vi "BeginTankDrive.vi"() -> (0 "error out":errorcluster)   [LabVIEW 2012]
uses:
  <vilib>/Rock Robotics/WPI/CAN/Jaguar/SubVIs/WPI_CANJaguar_SpeedReference.ctl
  <vilib>/Rock Robotics/WPI/CAN/Jaguar/SubVIs/WPI_CANJaguar_ControlMode.ctl
  <vilib>/Rock Robotics/WPI/MotorControl/WPI_MotorControlOpenCANJaguar.vi
  <vilib>/Rock Robotics/WPI/CAN/Jaguar/SubVIs/WPI_CANJaguar_BrakeCoastMode.ctl
panel:
  out "Succeeded?":bool
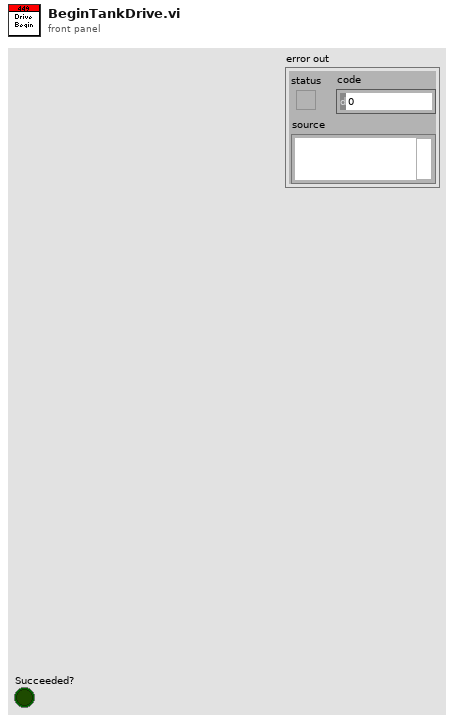
[diagram p1: front panel]
types:
  T1 = typedef "WPI_CANJaguar_ControlMode.ctl" = enum8{"Percent VBus", "Current", "Speed", "Position", "Voltage"}
  T2 = typedef "WPI_CANJaguar_SpeedReference.ctl" = u8
  T3 = typedef "WPI_MotorControlDeviceRef.ctl" = cluster{"DeviceStatus":errorcluster, "Type":enum16{"PWM", "CAN"}, "PWM":cluster{"Digital Module":T4, "PWM Channel":T5, "DeadBand":T6}, "CAN":cluster{"Device Number":u8, "Control Mode":T1, "Semaphore":T7, "Max Vout":dbl}, "Invert":bool, "TransformRef":T8, "InvTransformRef":T8}
  T4 = typedef "FPGA_TypedefDigitalModule.ctl" = enum16{"Digital Module 1", "Digital Module 2"}
  T5 = typedef "FPGA_DIOPWMChannel.ctl" = enum8{"PWM 1", "PWM 2", "PWM 3", "PWM 4", "PWM 5", "PWM 6", "PWM 7", "PWM 8", "PWM 9", "PWM 10", "Invalid"}
  T6 = typedef "WPI_PWMDeadband.ctl" = cluster{"Name":string, "maxPositivePwm":i32, "minPositivePwm":i32, "centerPwm":i32, "maxNegativePwm":i32, "minNegativePwm":i32, "angularRange":u16}
  T7 = typedef "Semaphore RefNum" = refnum<k1>
  T8 = typedef "WPI_PWMTransform_ConPane.ctl" = refnum<vi>
  T9 = typedef "WPI_CANJaguar_BrakeCoastMode.ctl" = enum8{"Jumper", "Brake", "Coast"}
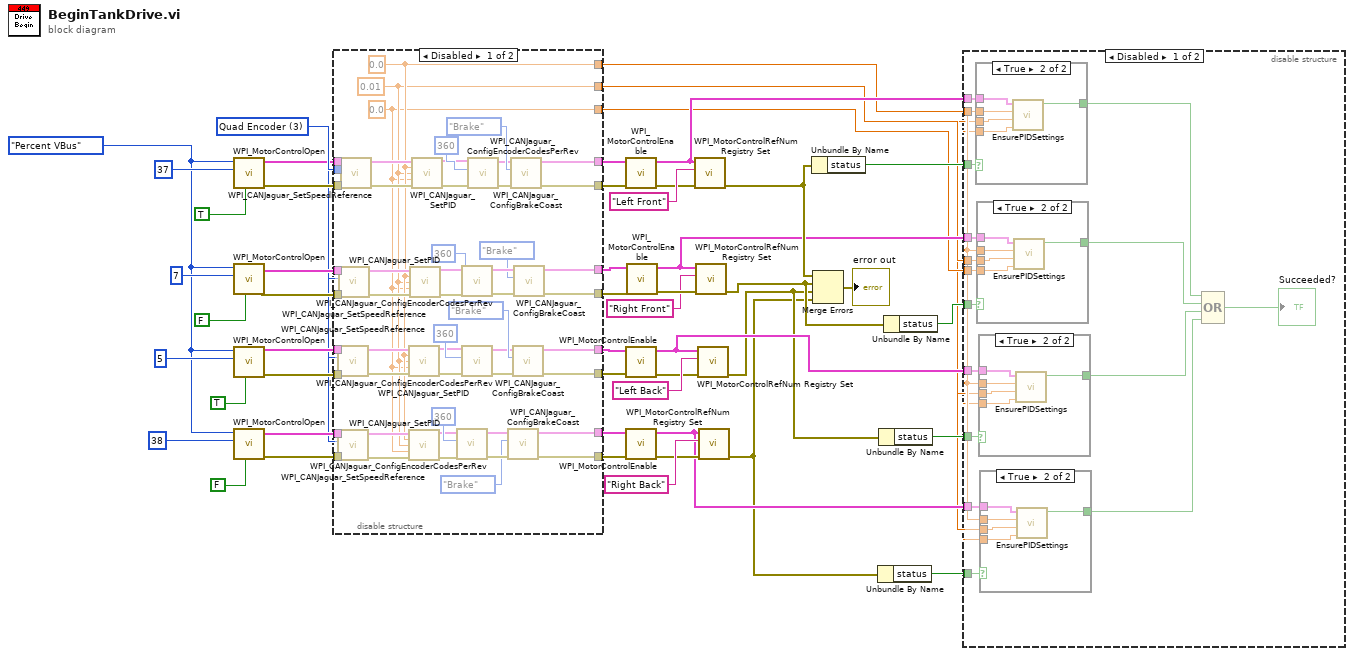
[diagram p0: block diagram]
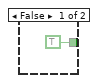
[diagram p2: hidden frame]
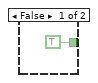
[diagram p3: hidden frame]
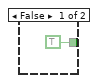
[diagram p4: hidden frame]
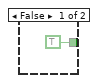
[diagram p5: hidden frame]
diagram:
  w39 = WPI_CANJaguar_ControlMode."Percent VBus" ("Control Mode")
  w42 = T2 3 items=["Encoder"=0, "Inv Encoder"=2, "Quad Encoder"=3, "None"=255] ("Speed Reference")
  n1 = call-poly <vilib>:"WPI_MotorControlOpen.vi"("Invert"=TRUE, "Device Number"=u8 37, "Control Mode"=w39) -> ("error out"=w37:errorcluster, "MotorControlDeviceRef"=w38:T3)  [unwired: 3 in, 4 out]
  n2 = call-poly <vilib>:"WPI_MotorControlOpen.vi"("Invert"=FALSE, "Device Number"=u8 7, "Control Mode"=w39) -> ("error out"=w19:errorcluster, "MotorControlDeviceRef"=w20:T3)  [unwired: 3 in, 4 out]
  n3 = call-poly <vilib>:"WPI_MotorControlOpen.vi"("Invert"=TRUE, "Device Number"=u8 5, "Control Mode"=w39) -> ("error out"=w44:errorcluster, "MotorControlDeviceRef"=w43:T3)  [unwired: 3 in, 4 out]
  n4 = call-poly <vilib>:"WPI_MotorControlOpen.vi"("Invert"=FALSE, "Device Number"=u8 38, "Control Mode"=w39) -> ("error out"=w45:errorcluster, "MotorControlDeviceRef"=w46:T3)  [unwired: 3 in, 4 out]
  n5 = disable-structure shown="Disabled" {
    disable-tunnel: w46 -> [w102 w104]
    disable-tunnel: w45 -> [w101 w103]
    disable-tunnel: w44 -> [w100 w105]
    disable-tunnel: w43 -> [w99 w106]
    disable-tunnel: w42 -> [w98 _]
    disable-tunnel: w38 -> [w95 w110]
    disable-tunnel: w37 -> [w94 w109]
    disable-tunnel: [w86 w110] -> w33
    disable-tunnel: [w85 w109] -> w32
    disable-tunnel: [w77 w105] -> w29
    disable-tunnel: [w76 w106] -> w28
    disable-tunnel: [w68 w104] -> w25
    disable-tunnel: [w67 w103] -> w24
    disable-tunnel: w20 -> [w63 w108]
    disable-tunnel: w19 -> [w62 w107]
    disable-tunnel: [w56 w107] -> w18
    disable-tunnel: [w55 w108] -> w17
    disable-tunnel: [w53 _] -> w10
    disable-tunnel: [w52 _] -> w9
    disable-tunnel: [w51 _] -> w8
    frame Disabled {
      w51 = 0.0 ("P")
      w52 = 0.01 ("P")
      w53 = 0.0 ("P")
      n6 = call <vilib>:"WPI_CANJaguar_SetSpeedReference.vi"("error in (no error)"=w100, "Speed Reference"=w98, "CAN Jaguar Ref"=w99) -> ("error out"=w84:errorcluster, "CAN Jaguar Ref Out"=w83:T3)  [unwired: 7 in]
      n7 = call <vilib>:"WPI_CANJaguar_SetSpeedReference.vi"("error in (no error)"=w101, "Speed Reference"=w98, "CAN Jaguar Ref"=w102) -> ("error out"=w75:errorcluster, "CAN Jaguar Ref Out"=w74:T3)  [unwired: 7 in]
      n8 = call <vilib>:"WPI_CANJaguar_SetSpeedReference.vi"("error in (no error)"=w62, "Speed Reference"=w98, "CAN Jaguar Ref"=w63) -> ("error out"=w65:errorcluster, "CAN Jaguar Ref Out"=w64:T3)  [unwired: 7 in]
      n9 = call <vilib>:"WPI_CANJaguar_SetSpeedReference.vi"("error in (no error)"=w94, "Speed Reference"=w98, "CAN Jaguar Ref"=w95) -> ("error out"=w92:errorcluster, "CAN Jaguar Ref Out"=w93:T3)  [unwired: 7 in]
      n10 = call <vilib>:"WPI_CANJaguar_SetPID.vi"("CAN Jaguar Ref"=w83, "P"=w53, "I"=w52, "D"=w51, "error in (no error)"=w84) -> ("CAN Jaguar Ref Out"=w78:T3, "error out"=w79:errorcluster)  [unwired: 9 in]
      n11 = call <vilib>:"WPI_CANJaguar_SetPID.vi"("CAN Jaguar Ref"=w74, "P"=w53, "I"=w52, "D"=w51, "error in (no error)"=w75) -> ("CAN Jaguar Ref Out"=w69:T3, "error out"=w70:errorcluster)  [unwired: 9 in]
      n12 = call <vilib>:"WPI_CANJaguar_SetPID.vi"("CAN Jaguar Ref"=w64, "P"=w53, "I"=w52, "D"=w51, "error in (no error)"=w65) -> ("CAN Jaguar Ref Out"=w57:T3, "error out"=w58:errorcluster)  [unwired: 9 in]
      n13 = call <vilib>:"WPI_CANJaguar_SetPID.vi"("CAN Jaguar Ref"=w93, "P"=w53, "I"=w52, "D"=w51, "error in (no error)"=w92) -> ("CAN Jaguar Ref Out"=w87:T3, "error out"=w88:errorcluster)  [unwired: 9 in]
      n14 = call <vilib>:"WPI_CANJaguar_ConfigEncoderCodesPerRev.vi"("error in (no error)"=w70, "Encoder Codes Per Rev"=u16 360, "CAN Jaguar Ref"=w69) -> ("error out"=w71:errorcluster, "CAN Jaguar Ref Out"=w72:T3)  [unwired: 7 in]
      n15 = call <vilib>:"WPI_CANJaguar_ConfigEncoderCodesPerRev.vi"("error in (no error)"=w58, "Encoder Codes Per Rev"=u16 360, "CAN Jaguar Ref"=w57) -> ("error out"=w59:errorcluster, "CAN Jaguar Ref Out"=w60:T3)  [unwired: 7 in]
      n16 = call <vilib>:"WPI_CANJaguar_ConfigEncoderCodesPerRev.vi"("error in (no error)"=w79, "Encoder Codes Per Rev"=u16 360, "CAN Jaguar Ref"=w78) -> ("error out"=w82:errorcluster, "CAN Jaguar Ref Out"=w81:T3)  [unwired: 7 in]
      n17 = call <vilib>:"WPI_CANJaguar_ConfigEncoderCodesPerRev.vi"("error in (no error)"=w88, "Encoder Codes Per Rev"=u16 360, "CAN Jaguar Ref"=w87) -> ("error out"=w89:errorcluster, "CAN Jaguar Ref Out"=w90:T3)  [unwired: 7 in]
      n18 = call <vilib>:"WPI_CANJaguar_ConfigBrakeCoast.vi"("error in (no error)"=w71, "Brake / Coast Mode"=WPI_CANJaguar_BrakeCoastMode."Brake", "CAN Jaguar Ref"=w72) -> ("error out"=w67:errorcluster, "CAN Jaguar Ref Out"=w68:T3)  [unwired: 7 in]
      n19 = call <vilib>:"WPI_CANJaguar_ConfigBrakeCoast.vi"("error in (no error)"=w89, "Brake / Coast Mode"=WPI_CANJaguar_BrakeCoastMode."Brake", "CAN Jaguar Ref"=w90) -> ("error out"=w85:errorcluster, "CAN Jaguar Ref Out"=w86:T3)  [unwired: 7 in]
      n20 = call <vilib>:"WPI_CANJaguar_ConfigBrakeCoast.vi"("error in (no error)"=w82, "Brake / Coast Mode"=WPI_CANJaguar_BrakeCoastMode."Brake", "CAN Jaguar Ref"=w81) -> ("error out"=w77:errorcluster, "CAN Jaguar Ref Out"=w76:T3)  [unwired: 7 in]
      n21 = call <vilib>:"WPI_CANJaguar_ConfigBrakeCoast.vi"("error in (no error)"=w59, "Brake / Coast Mode"=WPI_CANJaguar_BrakeCoastMode."Brake", "CAN Jaguar Ref"=w60) -> ("error out"=w56:errorcluster, "CAN Jaguar Ref Out"=w55:T3)  [unwired: 7 in]
    }
    frame Enabled {
    }
  }
  n22 = call <vilib>:"WPI_MotorControlEnable.vi"("error in (no error)"=w32, "CAN Jaguar Ref"=w33) -> ("error out"=w34:errorcluster, "CAN Jaguar Ref Out"=w15:T3)  [unwired: 1 in, 7 out]
  n23 = call <vilib>:"WPI_MotorControlEnable.vi"("error in (no error)"=w29, "CAN Jaguar Ref"=w28) -> ("error out"=w30:errorcluster, "CAN Jaguar Ref Out"=w12:T3)  [unwired: 1 in, 7 out]
  n24 = call <vilib>:"WPI_MotorControlEnable.vi"("error in (no error)"=w24, "CAN Jaguar Ref"=w25) -> ("error out"=w26:errorcluster, "CAN Jaguar Ref Out"=w11:T3)  [unwired: 1 in, 7 out]
  n25 = call <vilib>:"WPI_MotorControlEnable.vi"("error in (no error)"=w18, "CAN Jaguar Ref"=w17) -> ("error out"=w21:errorcluster, "CAN Jaguar Ref Out"=w13:T3)  [unwired: 1 in, 7 out]
  n26 = call <vilib>:"WPI_MotorControlRefNum Registry Set.vi"("error in (no error)"=w34, "refnum name"="Left Front", "MotorControlDevRef"=w15) -> ("error out"=w16:errorcluster)  [unwired: 8 out]
  n27 = call <vilib>:"WPI_MotorControlRefNum Registry Set.vi"("error in (no error)"=w21, "refnum name"="Right Front", "MotorControlDevRef"=w13) -> ("error out"=w7:errorcluster)  [unwired: 8 out]
  n28 = call <vilib>:"WPI_MotorControlRefNum Registry Set.vi"("error in (no error)"=w30, "refnum name"="Left Back", "MotorControlDevRef"=w12) -> ("error out"=w5:errorcluster)  [unwired: 8 out]
  n29 = call <vilib>:"WPI_MotorControlRefNum Registry Set.vi"("error in (no error)"=w26, "refnum name"="Right Back", "MotorControlDevRef"=w11) -> ("error out"=w3:errorcluster)  [unwired: 8 out]
  n30 = Unbundle By Name(w16) -> ("status"=w14:bool)
  n31 = Merge Errors(w16, w7, w5, w3) -> (→"error out":errorcluster)
  n32 = Unbundle By Name(w3) -> ("status"=w2:bool)
  n33 = Unbundle By Name(w5) -> ("status"=w4:bool)
  n34 = Unbundle By Name(w7) -> ("status"=w6:bool)
  n35 = disable-structure shown="Disabled" {
    disable-tunnel: w15 -> [w126 _]
    disable-tunnel: w14 -> [w125 _]
    disable-tunnel: w13 -> [w124 _]
    disable-tunnel: w12 -> [w123 _]
    disable-tunnel: w11 -> [w122 _]
    disable-tunnel: w10 -> [w121 _]
    disable-tunnel: w9 -> [w120 _]
    disable-tunnel: w8 -> [w119 _]
    disable-tunnel: w6 -> [w118 _]
    disable-tunnel: w4 -> [w117 _]
    disable-tunnel: w2 -> [w116 _]
    frame Disabled {
      n36 = case shown="True" w125 {
        tunnel: w126 -> [_ w150]
        tunnel: w121 -> [_ w149]
        tunnel: w120 -> [_ w148]
        tunnel: w119 -> [_ w147]
        tunnel: [TRUE ("Succeeded?") w146] -> w115
        frame False {
        }
        frame True {
          n37 = call "EnsurePIDSettings.vi"("D"=w147, "I"=w148, "P"=w149, "CAN Jaguar Ref"=w150) -> ("Succeeded?"=w146:bool)  [unwired: 7 in]
        }
      }
      n38 = case shown="True" w118 {
        tunnel: w124 -> [_ w144]
        tunnel: w121 -> [_ w143]
        tunnel: w120 -> [_ w142]
        tunnel: w119 -> [_ w141]
        tunnel: [TRUE ("Succeeded?") w140] -> w114
        frame False {
        }
        frame True {
          n39 = call "EnsurePIDSettings.vi"("D"=w141, "I"=w142, "P"=w143, "CAN Jaguar Ref"=w144) -> ("Succeeded?"=w140:bool)  [unwired: 7 in]
        }
      }
      n40 = case shown="True" w117 {
        tunnel: w123 -> [_ w138]
        tunnel: w121 -> [_ w137]
        tunnel: w120 -> [_ w136]
        tunnel: w119 -> [_ w135]
        tunnel: [TRUE ("Succeeded?") w134] -> w112
        frame False {
        }
        frame True {
          n41 = call "EnsurePIDSettings.vi"("D"=w135, "I"=w136, "P"=w137, "CAN Jaguar Ref"=w138) -> ("Succeeded?"=w134:bool)  [unwired: 7 in]
        }
      }
      n42 = case shown="True" w116 {
        tunnel: w122 -> [_ w132]
        tunnel: w121 -> [_ w131]
        tunnel: w120 -> [_ w130]
        tunnel: w119 -> [_ w129]
        tunnel: [TRUE ("Succeeded?") w128] -> w113
        frame False {
        }
        frame True {
          n43 = call "EnsurePIDSettings.vi"("D"=w129, "I"=w130, "P"=w131, "CAN Jaguar Ref"=w132) -> ("Succeeded?"=w128:bool)  [unwired: 7 in]
        }
      }
      n44 = Compound Arithmetic op=OR(w115, w114, w112, w113) -> (→"Succeeded?":bool)
    }
    frame Enabled {
    }
  }
